vi "327_sound_output_template.vi"() -> ()   [LabVIEW 2019]
doc: "This VI illustrates how to generate and play sine, square, sawtooth and triangle waveforms. You can change the frequency and type of the waveform generated as it plays continuously."
uses:
  <vilib>/sound2/lvsound2.llb/Sound Data Format.ctl
  <vilib>/sound2/lvsound2.llb/Sampling Mode.ctl
  <vilib>/sound2/lvsound2.llb/Sound Output Set Volume (Single).vi
  <vilib>/sound2/lvsound2.llb/Sound Output Write (DBL Single).vi
  <vilib>/measure/NI_MABase.lvlib
panel:
  in  "signal type":T1(ring)
  in  "signal frequency control":dbl(knob)=100.1 step=0.1 scale=0.0..200.0 scale format="%#_3f"
  in  "Sound Format":T2={"sample rate (S/s)"=11025.0, "number of channels"=2, "bits per sample"=16}
  in  "Volume":dbl(slide)=62.244897959183675 scale=0.0..100.0
  out "Generated Sound":waveform(dbl)(graph)={"t0"=timestamp(14.058956916099774 s since 1904-01-01), "dt"=9.070294784580499e-05, "Y"=array[5000 elements]}
  in  "stop":bool
  in  "Samples/ch":i32=5000
  in  "Device ID":u32
  # "Configuration"
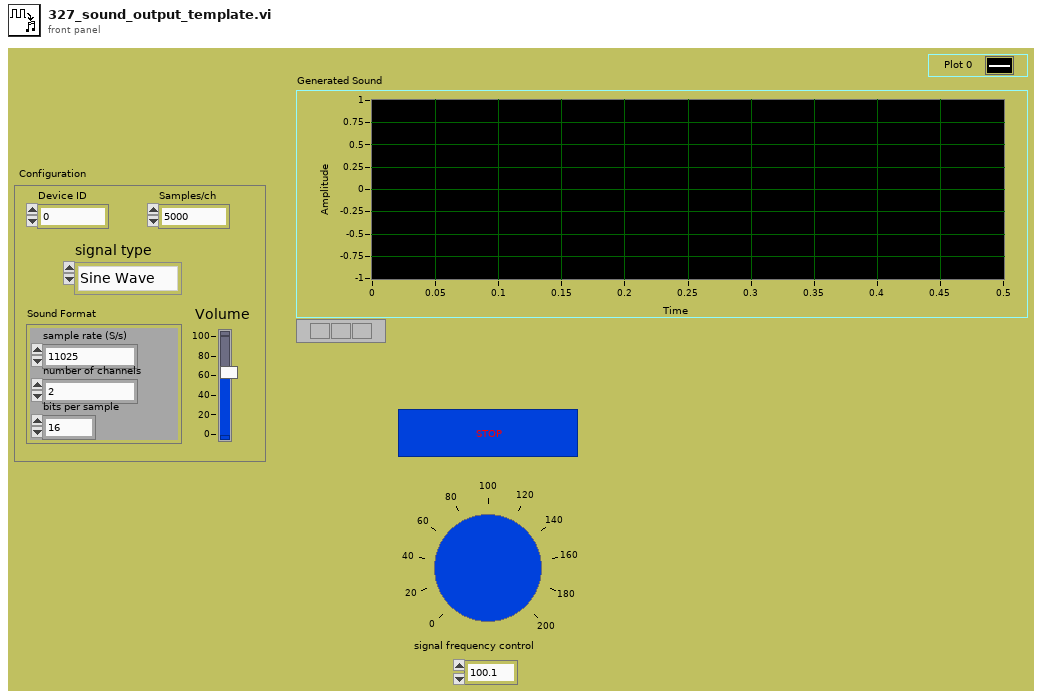
[diagram p1: front panel]
types:
  T1 = enum16{"Sine Wave", "Triangle Wave", "Square Wave", "Sawtooth Wave"}
  T2 = typedef "Sound Data Format.ctl" = cluster{"sample rate (S/s)":dbl, "number of channels":i32, "bits per sample":i32}
  T3 = typedef "Sampling Mode.ctl" = i32
  T4 = typedef "Sound Output Task ID.ctl" = u32
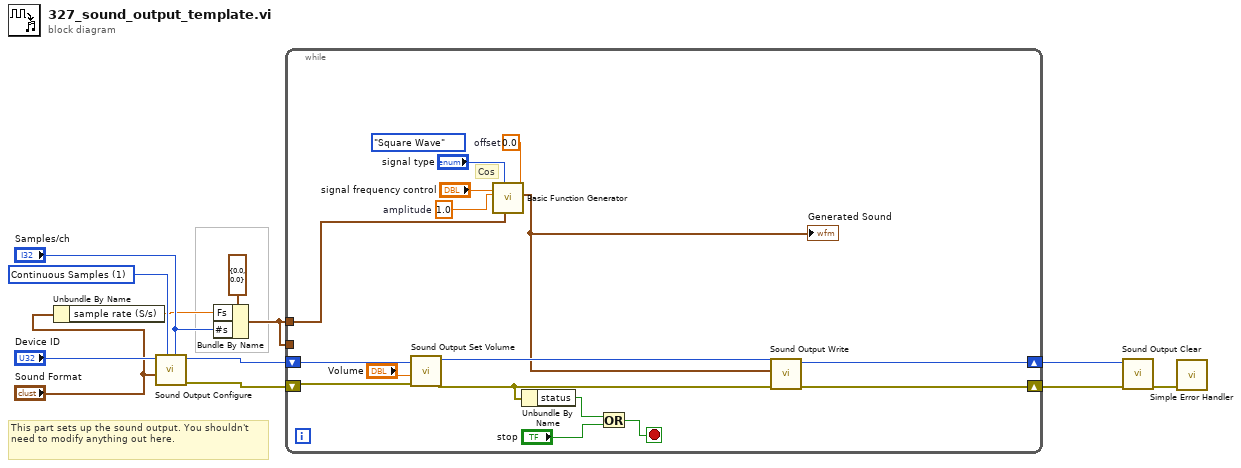
[diagram p0: block diagram]
diagram:
  w7 = T3 1 items=["Finite Samples", "Continuous Samples"] ("sample mode")
  # "This part sets up the sound output. You shouldn't need to modify anything out here."
  n1 = Unbundle By Name("Sound Format") -> ("sample rate (S/s)"=w2:dbl)
  n2 = call <vilib>:"Sound Output Configure.vi"("number of samples/ch"="Samples/ch", "sample mode"=w7, "sound format"="Sound Format", "device ID"="Device ID") -> ("error out"=w12:errorcluster, "task ID"=w11:T4)  [unwired: 6 in]
  n3 = Bundle By Name(cluster=cluster{"Fs":dbl, "#s":dbl} {"Fs"=0.0, "#s"=0.0} ("sampling info"), "Fs"=w2, "#s"="Samples/ch") -> (w1:cluster{"Fs":dbl, "#s":dbl})
  n4 = while {
    shift-right: [w27] -> w10
    shift-left: w12 -> [w22]
    shift-right: [w28] -> w9
    shift-left: w11 -> [w20]
    tunnel: w1 -> [w13]
    tunnel: w1 -> [_]
    stop <- w25 stop-if-true
    (unwired) T1."Square Wave" ("signal type")
    w15 = 0.0  # offset
    w17 = 1.0  # amplitude
    # "Cos"
    n5 = call-poly <vilib>:"Sound Output Set Volume.vi"("error in (no error)"=w22, "volume"="Volume", "task ID"=w20) -> ("error out"=w23:errorcluster, "task ID out"=w21:T4)  [unwired: 7 in]
    n6 = call <vilib>:"Basic Function Generator.vi"("offset"=w15, "sampling info"=w13, "signal type"="signal type", "amplitude"=w17, "frequency"="signal frequency control") -> ("signal out"=w14:waveform(dbl))  [unwired: 4 in, 2 out]
    "Generated Sound" <- w14
    n7 = Unbundle By Name(w23) -> ("status"=w24:bool)
    n8 = Or(x=w24, y="stop") -> (x .or. y?=w25:bool)
    n9 = call-poly <vilib>:"Sound Output Write.vi"("error in (no error)"=w23, "data"=w14, "task ID"=w21) -> ("error out"=w27:errorcluster, "task ID out"=w28:T4)  [unwired: 7 in]
  }
  n10 = call <vilib>:"Sound Output Clear.vi"("error in (no error)"=w10, "task ID"=w9) -> ("error out"=w4:errorcluster)  [unwired: 9 in]
  n11 = call <vilib>:"Simple Error Handler.vi"("error in (no error)"=w4) -> ()  [unwired: 4 in, 5 out]
